vi "ArduinoMenuFacade.vi"(0 "Data In":T4, 2 "Display State In":T2, 3 "Container State":T3) -> (6 "Data Out":T4, 7 "Display State Out":T2, 8 "Action":T1)   [LabVIEW 2020, in "ArduinoMenuXControl.xctl"]
uses:
  ArduinoMenuXControl.xctl
  ArduinoMenuData.ctl
  <vilib>/_xctls/Container State.ctl
  ArduinoMenuState.ctl
  <vilib>/_xctls/Action.ctl
  <vilib>/_xctls/XControlSupport.lvlib
panel:
  in  "Board":u16(ring)
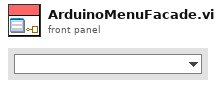
[diagram p1: front panel]
types:
  T1 = typedef "XControlSupport.lvlib/Action.ctl" = cluster{"Data Changed?":bool, "State Changed?":bool, "Action Name":string}
  T2 = typedef "ArduinoMenuXControl.xctl/ArduinoMenuState.ctl" = cluster{"Numeric":dbl}
  T3 = typedef "XControlSupport.lvlib/Container State.ctl" = cluster{"Indicator?":bool, "Run Mode?":bool, " Refnum":refnum<vi>}
  T4 = typedef "ArduinoMenuXControl.xctl/ArduinoMenuData.ctl" = string
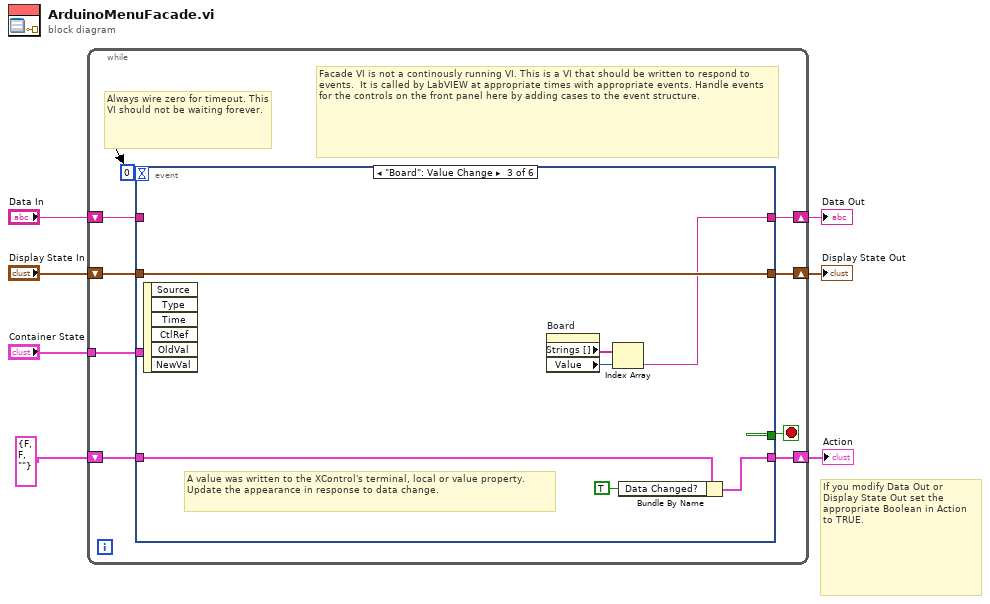
[diagram p0: block diagram]
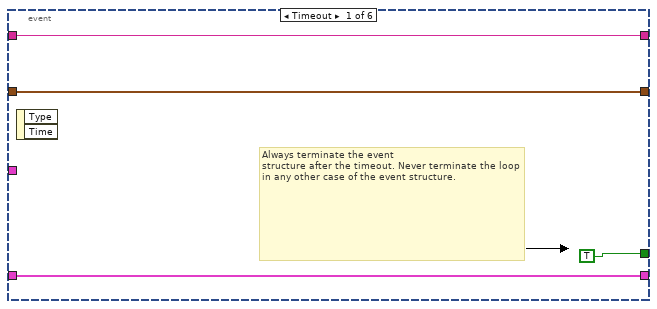
[diagram p2: hidden frame]
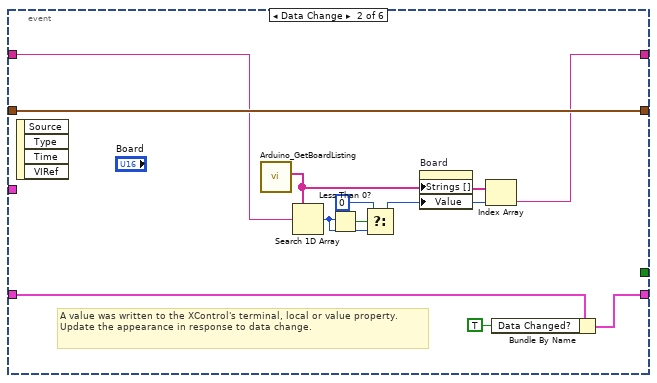
[diagram p3: hidden frame]
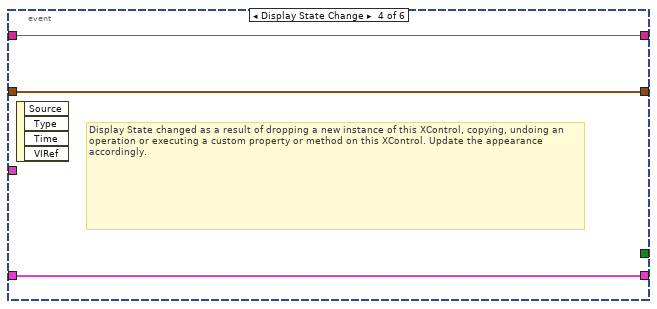
[diagram p4: hidden frame]
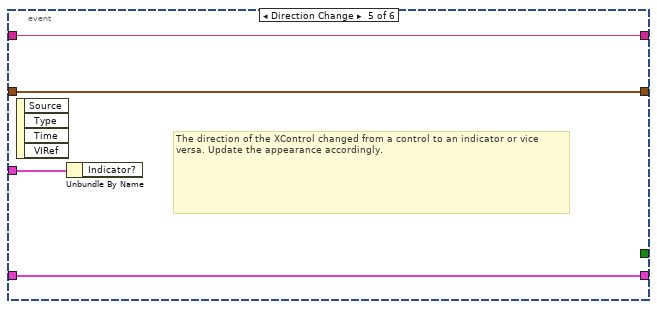
[diagram p5: hidden frame]
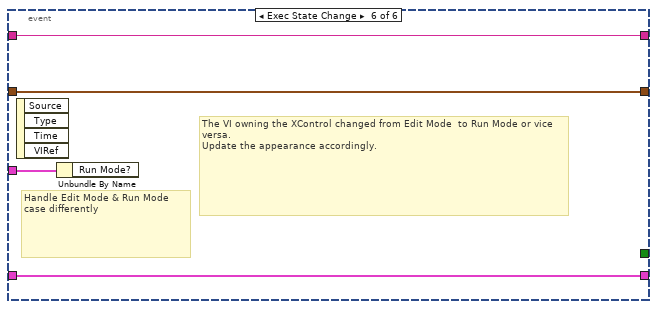
[diagram p6: hidden frame]
diagram:
  # "If you modify Data Out or\nDisplay State Out set the\nappropriate Boolean in Action\nto TRUE."
  n1 = while {
    shift-right: [w15] -> w4
    shift-left: "Display State In" -> [w16]
    tunnel: "Container State" -> [w12]
    shift-right: [w10] -> w7
    shift-left: "Data In" -> [w11]
    shift-right: [w8] -> w2
    shift-left: T1 {"Data Changed?"=FALSE, "State Changed?"=FALSE, "Action Name"=""} ("Action") -> [w9]
    stop <- w14 stop-if-true
    # "Facade VI is not a continously running VI. This is a VI that should be written to respond to events.  It is called by LabVIEW at appropriate times with appropriate events. Handle events for the controls on the front panel here by adding cases to the event structure."
    # "Always wire zero for timeout. This\nVI should not be waiting forever."
    n2 = event shown="[2] \"Board\": Value Change" {
      selector: _ -> [_ _ _ _ _ _]
      dyn-events: _ -> [_ _ _ _ _ _]
      timeout: 0 -> [_ _ _ _ _ _]
      tunnel: w16 -> [w18 w31 w38 w41 w44 w48]
      tunnel: [w18 w31 w38 w41 w44 w48] -> w15
      tunnel: [TRUE _ _ _ _ _] -> w14
      tunnel: w12 -> [_ _ _ _ w45 w49]
      tunnel: w11 -> [w17 w24 _ w40 w43 w47]
      tunnel: [w17 w25 w37 w40 w43 w47] -> w10
      tunnel: [w19 w23 w36 w39 w42 w46] -> w8
      tunnel: w9 -> [w19 w22 w35 w39 w42 w46]
      event Timeout {
        # "Always terminate the event\nstructure after the timeout. Never terminate the loop in any other case of the event structure."
        n3 = event-data() -> ()  [unwired: 1 in, 2 out]
      }
      event Data Change {
        # "A value was written to the XControl's terminal, local or value property.\nUpdate the appearance in response to data change."
        n4 = event-data() -> ()  [unwired: 1 in, 4 out]
        n5 = call "Arduino_GetBoardListing.vi"() -> ("All Names"=w27:string[])  [unwired: 11 in]
        n6 = Search 1D Array(1D array=w27, element=w24) -> (index of element=w29:i32)  [unwired: 1 in]
        n7 = Less Than 0?(x=w29) -> (x < 0?=w30:bool)
        n8 = Select(t=0, s=w30, f=w29) -> (s? t:f=w26:i32)
        n9 = property on="Board" class="Ring (strict)"("Strings []"=w27, "Value"=w26) -> ()  [unwired: 2 in, 2 out]
        n10 = Index Array(array=w27, index=w26) -> (element=w25:string)
        n11 = Bundle By Name(cluster=w22, "Data Changed?"=TRUE) -> (w23:T1)
      }
      event "Board": Value Change {
        # "A value was written to the XControl's terminal, local or value property.\nUpdate the appearance in response to data change."
        n12 = event-data() -> ()  [unwired: 1 in, 6 out]
        n13 = property on="Board" class="Ring (strict)"() -> ("Strings []"=w32:string[], "Value"=w33:u16)  [unwired: 2 in, 2 out]
        n14 = Index Array(array=w32, index=w33) -> (element=w37:string)
        n15 = Bundle By Name(cluster=w35, "Data Changed?"=TRUE) -> (w36:T1)
      }
      event Display State Change {
        # "Display State changed as a result of dropping a new instance of this XControl, copying, undoing an operation or executing a custom property or method on this XControl. Update the appearance accordingly."
        n16 = event-data() -> ()  [unwired: 1 in, 4 out]
      }
      event Direction Change {
        # "The direction of the XControl changed from a control to an indicator or vice versa. Update the appearance accordingly."
        n17 = event-data() -> ()  [unwired: 1 in, 4 out]
        n18 = Unbundle By Name(w45) -> ()  [unwired: 1 out]
      }
      event Exec State Change {
        # "The VI owning the XControl changed from Edit Mode  to Run Mode or vice versa.\nUpdate the appearance accordingly."
        # "Handle Edit Mode & Run Mode\ncase differently"
        n19 = event-data() -> ()  [unwired: 1 in, 4 out]
        n20 = Unbundle By Name(w49) -> ()  [unwired: 1 out]
      }
    }
  }
  "Display State Out" <- w4
  "Data Out" <- w7
  "Action" <- w2
